vi "ListFiles.vi"(11 "Folder":path) -> ()   [LabVIEW 2019]
panel:
  out "All Files in Dir":path[](array[path])
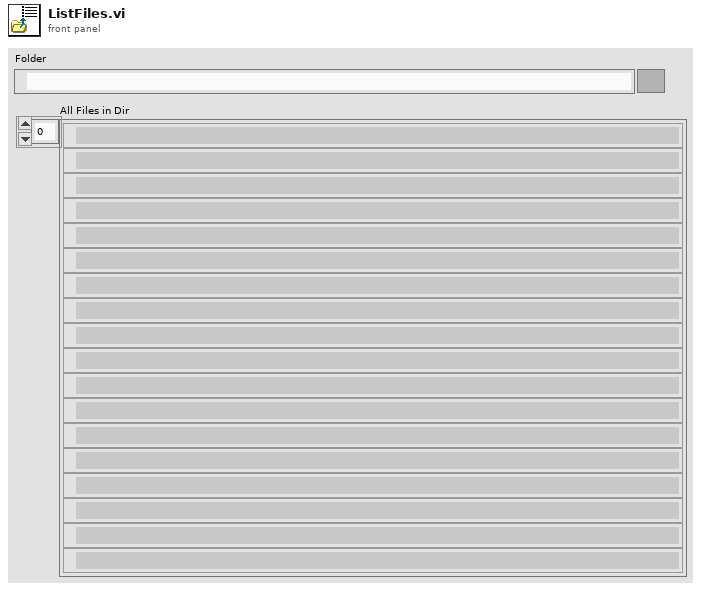
[diagram p1: front panel]
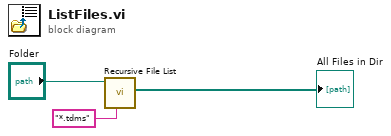
[diagram p0: block diagram]
diagram:
  n1 = call <vilib>:"Recursive File List.vi"("pattern"="*.tdms", "Folder Path"="Folder") -> ("All Files in Dir"=→"All Files in Dir":path[])  [unwired: 5 in, 4 out]
